vi "dfd_DFXPSimu Casting (vector).vi"(5 "quantize output? (T)":bool=TRUE, 7 "op params":T3={"source"=0, "is floating?"=FALSE, "o-mode"=enum."Wrap", "q-mode"=enum."Truncation", "wl"=1, "high limit"=0, "low limit"=0, "iwl"=0, "sign?"=TRUE} {"source" items=["Coef a/k"=0, "Coef b/v"=7, "Input"=1, "Output"=2, "Multiplicand"=3, "Product"=4, "Sum"=5, "Delay"=6, "Gain"=8]}, 8 "filtering statistics in":T7(array[cluster]) {"statistics information"."min value" format="%.2f"; "statistics information"."max value" format="%.2f"; "Quantizer Source" items=["Coefficients a/k"=0, "Coefficients b/v"=7, "Input"=1, "Output"=2, "Multiplicand"=3, "Product"=4, "Sum"=5, "Delay"=6]}, 11 "Value in":T8 {"High 64" format="%.0x"; "Low 64" format="%.0x"}) -> (0 "filtering statistics out":T7(array[cluster]) {"statistics information"."min value" format="%.2f"; "statistics information"."max value" format="%.2f"; "Quantizer Source" items=["Coefficients a/k"=0, "Coefficients b/v"=7, "Input"=1, "Output"=2, "Multiplicand"=3, "Product"=4, "Sum"=5, "Delay"=6]}, 3 "Value out":T2)   [LabVIEW 2017, in "NI_DigFilter_FXP.lvlib"]
uses:
  <vilib>/addons/Digital Filter Design/NI_DigFilter_FXP.lvlib
  <vilib>/addons/Digital Filter Design/_Objects.llb/dfd_DFXP Data Type 128bits (vector).ctl
  <vilib>/addons/Digital Filter Design/_Objects.llb/dfd_DFXP Data Type (vector).ctl
  <vilib>/addons/Digital Filter Design/_Objects.llb/DFD Quantization Sources.ctl
  <vilib>/addons/Digital Filter Design/_Objects.llb/DFD FXP Statistics Data.ctl
  <vilib>/addons/Digital Filter Design/_Objects.llb/dfd_DFXP Operation Parameter.ctl
  <vilib>/addons/Digital Filter Design/_Objects.llb/dfd_Internal Quantization Srcs.ctl
  <vilib>/addons/Digital Filter Design/_Objects.llb/dfd_DFXP Data Type 128bits (scaler).ctl
  <vilib>/addons/Digital Filter Design/NI_DigFilterLicensed.lvlib
panel:
  in  "Value type":T1 {"Low 64" format="%.0x"; "High 64" format="%.0x"}
  in  "Value out type":T2
  in  "Value out type":T2
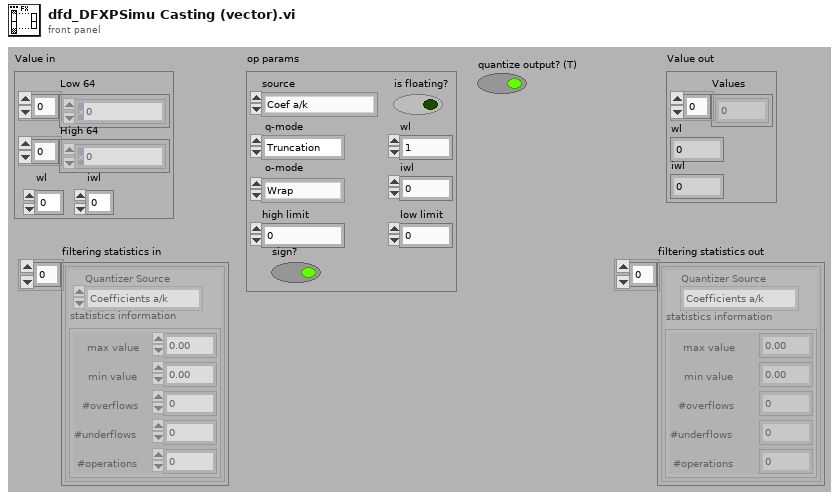
[diagram p1: front panel]
types:
  T1 = typedef "dfd_DFXP Data Type 128bits (scaler).ctl" = cluster{"Low 64":u64, "High 64":i64, "wl":i16, "iwl":i16}
  T2 = typedef "dfd_DFXP Data Type (vector).ctl" = cluster{"Values":i64[], "wl":i16, "iwl":i16}
  T3 = typedef "dfd_DFXP Operation Parameter.ctl" = cluster{"source":T4, "is floating?":bool, "o-mode":enum16{"Saturation", "Wrap"}, "q-mode":enum16{"Nearest", "Truncation"}, "wl":i16, "high limit":i64, "low limit":i64, "iwl":i16, "sign?":bool}
  T4 = typedef "NI_DigFilterLicensed.lvlib/dfd_Internal Quantization Srcs.ctl" = u16
  T5 = typedef "NI_DigFilterLicensed.lvlib/DFD Quantization Sources.ctl" = u16
  T6 = typedef "NI_DigFilterLicensed.lvlib/DFD FXP Statistics Data.ctl" = cluster{"max value":ext, "min value":ext, "#overflows":i32, "#underflows":i32, "#operations":i32}
  T7 = cluster{"Quantizer Source":T5, "statistics information":T6}[]
  T8 = typedef "dfd_DFXP Data Type 128bits (vector).ctl" = cluster{"Low 64":u64[], "High 64":i64[], "wl":i16, "iwl":i16}
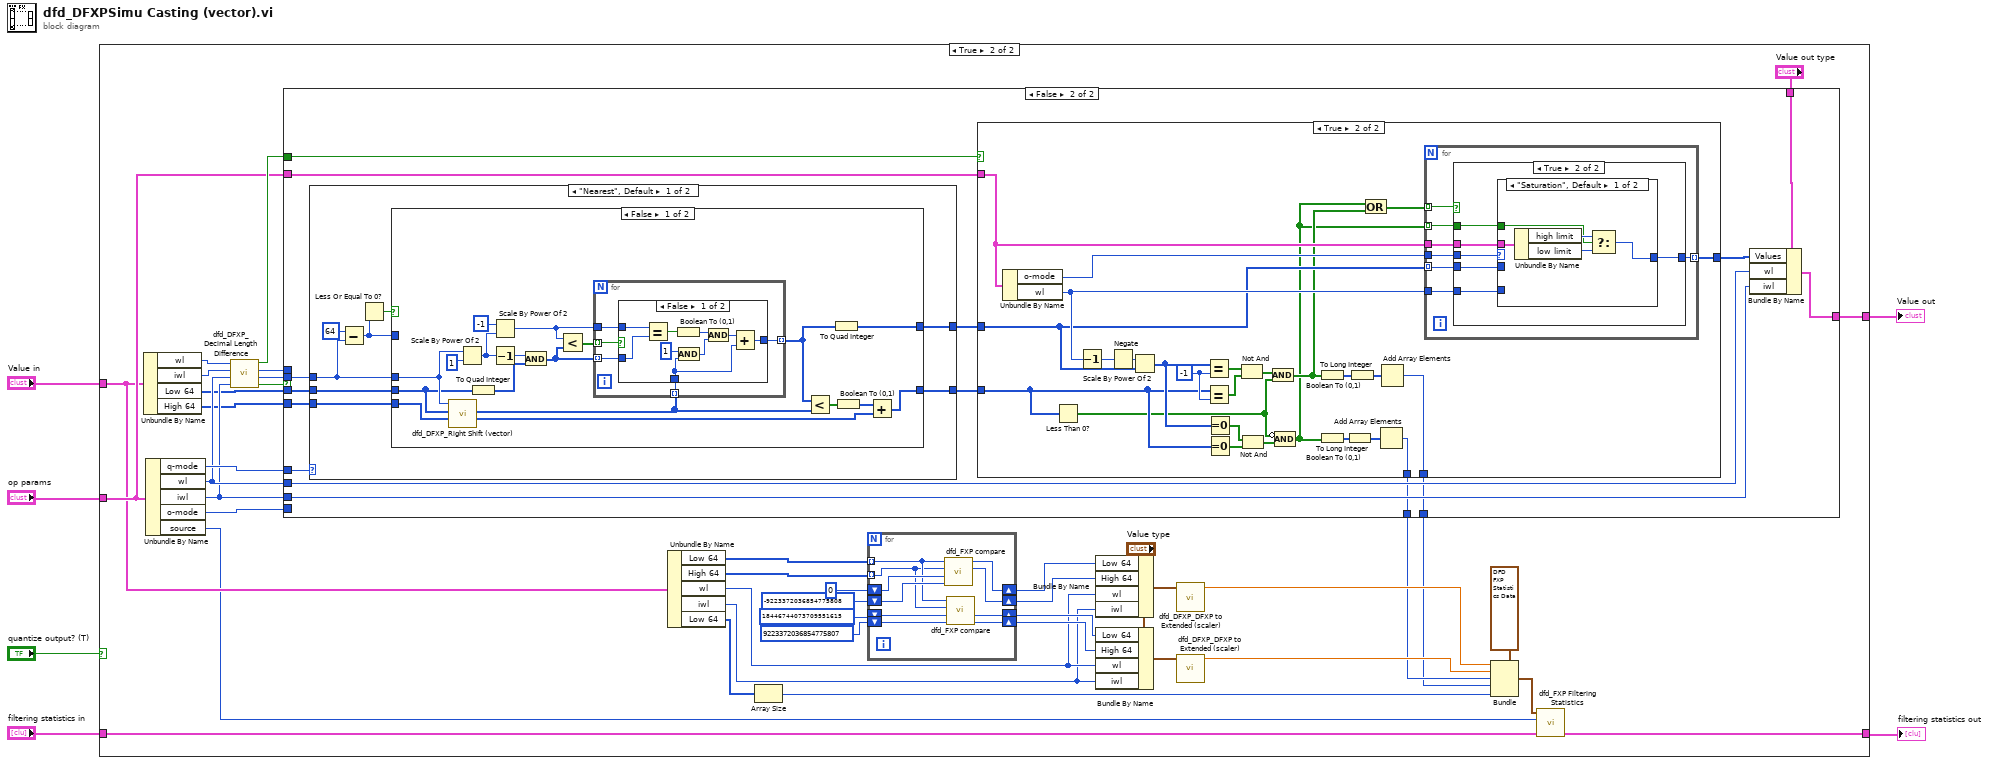
[diagram p0: block diagram]
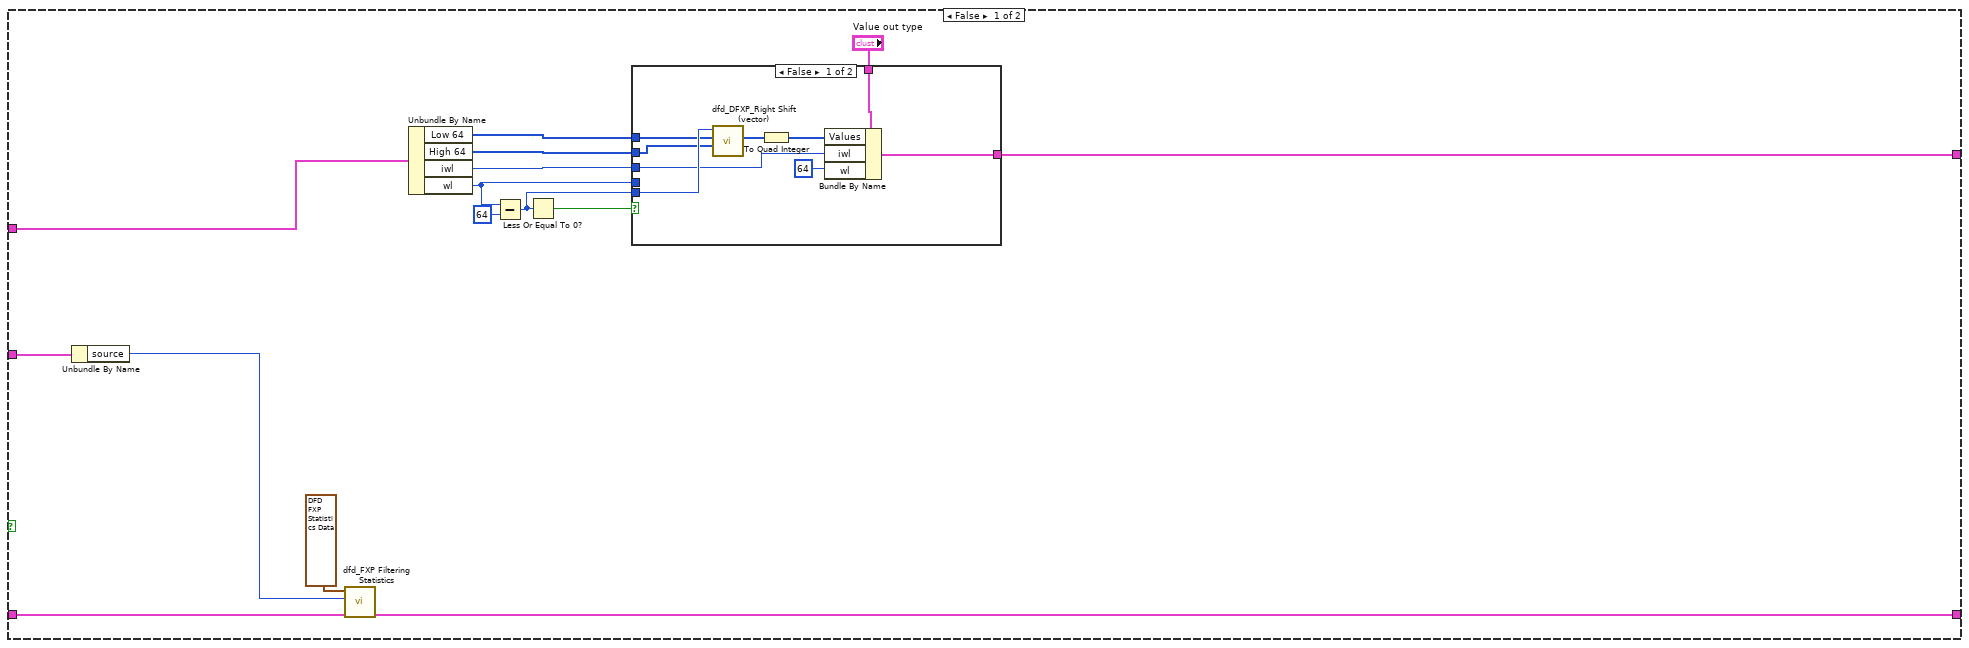
[diagram p2: hidden frame]
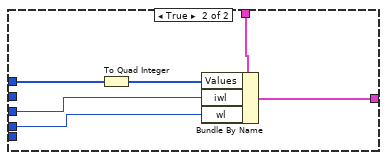
[diagram p3: hidden frame]
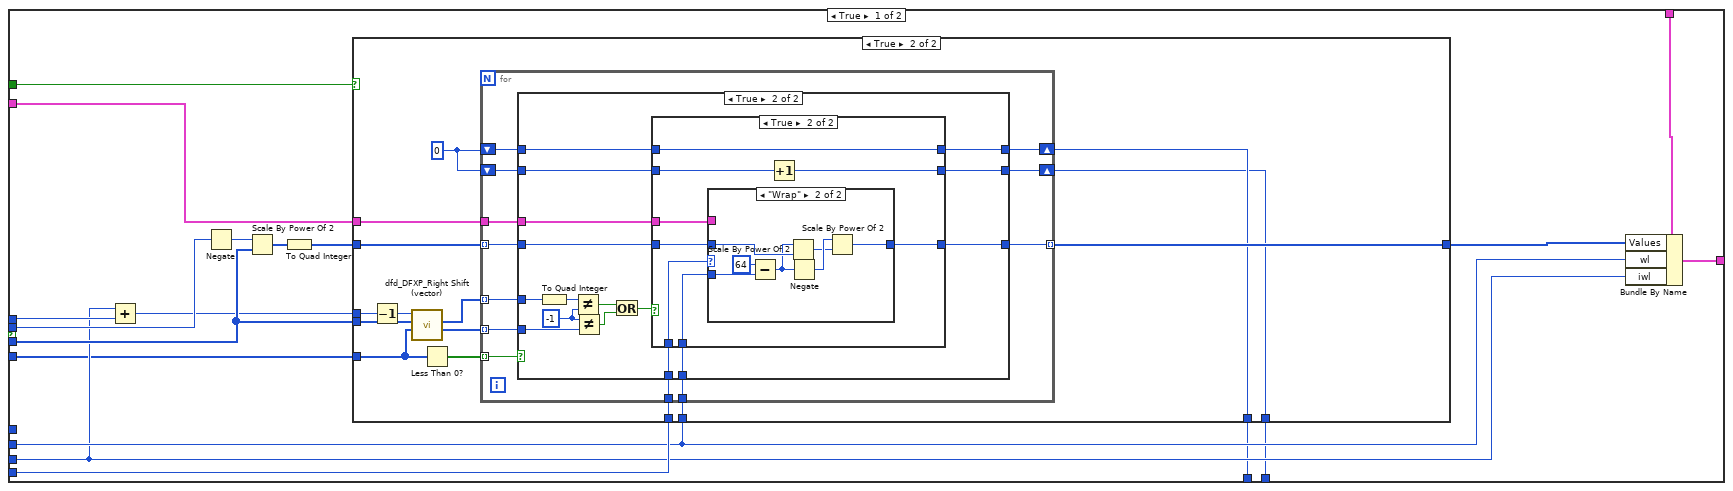
[diagram p4: hidden frame]
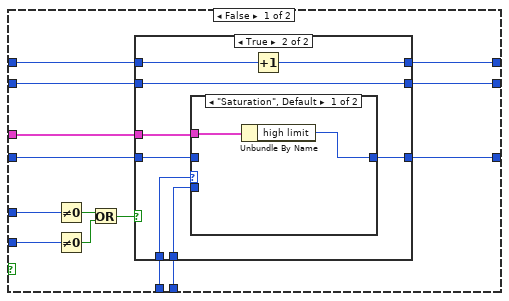
[diagram p6: hidden frame]
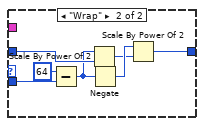
[diagram p8: hidden frame]
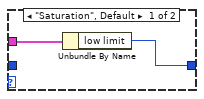
[diagram p10: hidden frame]
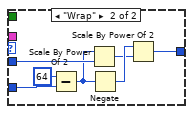
[diagram p13: hidden frame]
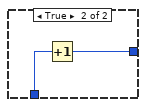
[diagram p14: hidden frame]
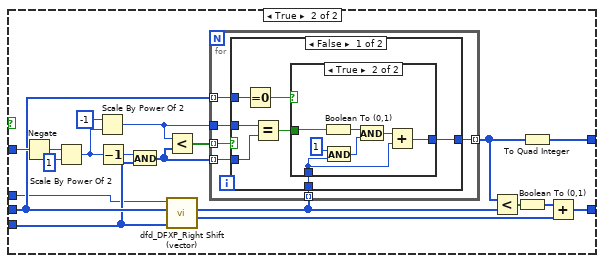
[diagram p15: hidden frame]
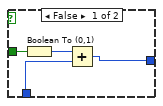
[diagram p16: hidden frame]
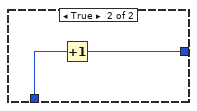
[diagram p17: hidden frame]
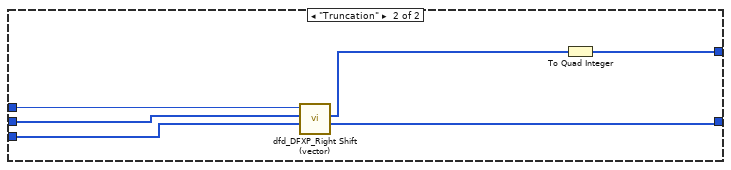
[diagram p18: hidden frame]
diagram:
  n1 = case shown="True" "quantize output? (T)" {
    tunnel: [w12 w67] -> w1
    tunnel: "op params" -> [w21 w70]
    tunnel: "Value in" -> [w13 w63]
    tunnel: "filtering statistics in" -> [w8 w45]
    tunnel: [w7 w37] -> w6
    frame False {
      n2 = Unbundle By Name(w21) -> ("source"=w10:T4)
      n3 = call <vilib>:"dfd_FXP Filtering Statistics.vi"("filtering statistics in"=w8, "source"=w10, "new data"=T6 {"max value"=-inf, "min value"=inf, "#overflows"=0, "#underflows"=0, "#operations"=1}) -> ("filtering statistics out"=w7:T7)  [unwired: 8 in]
      n4 = Unbundle By Name(w13) -> ("Low 64"=w19:u64[], "High 64"=w17:i64[], "iwl"=w18:i16, "wl"=w15:i16)
      n5 = Subtract(x=w15, y=i16 64) -> (x-y=w16:i16)
      n6 = Less Or Equal To 0?(x=w16) -> (x <= 0?=w11:bool)
      n7 = case shown="False" w11 {
        tunnel: w19 -> [w29 w36]
        tunnel: w18 -> [w25 w34]
        tunnel: [w23 w33] -> w12
        tunnel: w17 -> [w28 _]
        tunnel: w16 -> [w30 _]
        tunnel: w15 -> [_ w32]
        tunnel: "Value out type" -> [w22 w31]
        frame False {
          n8 = call <vilib>:"dfd_DFXP_Right Shift (vector).vi"("High 64"=w28, "Low 64"=w29, "Num"=w30) -> ("Low 64"=w26:u64[])  [unwired: 8 out]
          n9 = To Quad Integer(1:w26) -> (0:w27:i64[])
          n10 = Bundle By Name(cluster=w22, "Values"=w27, "iwl"=w25, "wl"=i16 64) -> (w23:T2)
        }
        frame True {
          n11 = To Quad Integer(1:w36) -> (0:w35:i64[])
          n12 = Bundle By Name(cluster=w31, "Values"=w35, "iwl"=w34, "wl"=w32) -> (w33:T2)
        }
      }
    }
    frame True {
      n13 = Unbundle By Name(w63) -> ("wl"=w76:i16, "iwl"=w77:i16, "Low 64"=w66:u64[], "High 64"=w65:i64[])
      n14 = Unbundle By Name(w70) -> ("q-mode"=w78:enum16{"Nearest", "Truncation"}, "wl"=w71:i16, "iwl"=w69:i16, "o-mode"=w72:enum16{"Saturation", "Wrap"}, "source"=w62:T4)
      n15 = call <vilib>:"dfd_DFXP_Decimal Length Difference.vi"("iwl 2"=w69, "wl 2"=w71, "iwl 1"=w77, "wl 1"=w76) -> ("fwl_diff <= 0?"=w75:bool, "fwl_diff"=w73:i16, "fwl"=w64:i16, "iwl_diff >= 0?"=w74:bool)  [unwired: 4 out]
      n16 = case shown="False" w75 {
        tunnel: w78 -> [_ w219]
        tunnel: w66 -> [w97 w218]
        tunnel: w70 -> [w105 w214]
        tunnel: w74 -> [w98 w216]
        tunnel: w73 -> [w96 w215]
        tunnel: w72 -> [w104 _]
        tunnel: w71 -> [w100 w211]
        tunnel: [w99 w209] -> w67
        tunnel: w69 -> [w93 w210]
        tunnel: "Value out type" -> [w102 w213]
        tunnel: w65 -> [w91 w208]
        tunnel: w64 -> [w94 _]
        tunnel: [w90 w206] -> w41
        tunnel: [w89 w205] -> w40
        frame True {
          n17 = Add(x=w93, y=w94) -> (x+y=w92:i16)
          n18 = Negate(x=w96) -> (-x=w106:i16)
          n19 = Scale By Power Of 2(n=w106, x=w97) -> (x*2^n=w103:u64[])
          n20 = To Quad Integer(1:w103) -> (0:w95:i64[])
          n21 = case shown="True" w98 {
            tunnel: w105 -> [_ w115]
            tunnel: w104 -> [_ w114]
            tunnel: w95 -> [w107 w113]
            tunnel: [w107 w111] -> w101
            tunnel: w100 -> [_ w112]
            tunnel: w97 -> [_ w121]
            tunnel: [_ w109] -> w90
            tunnel: [_ w108] -> w89
            tunnel: w92 -> [_ w122]
            tunnel: w91 -> [_ w120]
            frame False {
            }
            frame True {
              w110 = 0 ("high limit")
              n22 = Decrement(x=w122) -> (x-1=w117:i16)
              n23 = call <vilib>:"dfd_DFXP_Right Shift (vector).vi"("High 64"=w120, "Low 64"=w121, "Num"=w117) -> ("High 64"=w118:i64[], "Low 64"=w119:u64[])  [unwired: 7 out]
              n24 = Less Than 0?(x=w120) -> (x < 0?=w116:bool[])
              n25 = for {
                tunnel: w119 -> [w134] mode=indexing
                tunnel: w118 -> [w133] mode=indexing
                tunnel: w116 -> [w132] mode=indexing
                tunnel: w115 -> [w131]
                tunnel: w114 -> [w130]
                tunnel: w113 -> [w129] mode=indexing
                tunnel: w112 -> [w128]
                tunnel: [w127] -> w111 mode=indexing
                shift-right: [w125] -> w109
                shift-left: w110 -> [w126]
                shift-right: [w123] -> w108
                shift-left: w110 -> [w124]
                n26 = case shown="True" w132 {
                  tunnel: w134 -> [w148 w181]
                  tunnel: w133 -> [w147 w180]
                  tunnel: w131 -> [w143 w173]
                  tunnel: w130 -> [w142 w170]
                  tunnel: w129 -> [w141 w172]
                  tunnel: w128 -> [w140 w171]
                  tunnel: [w139 w169] -> w127
                  tunnel: w126 -> [w138 w177]
                  tunnel: [w137 w175] -> w125
                  tunnel: w124 -> [w136 w176]
                  tunnel: [w135 w174] -> w123
                  frame False {
                    n27 = Not Equal To 0?(x=w148) -> (x != 0?=w146:bool)
                    n28 = Not Equal To 0?(x=w147) -> (x != 0?=w145:bool)
                    n29 = Or(x=w146, y=w145) -> (x .or. y?=w144:bool)
                    n30 = case shown="True" w144 {
                      tunnel: [w151 w159] -> w139
                      tunnel: w141 -> [w151 w158]
                      tunnel: w143 -> [_ w157]
                      tunnel: w142 -> [_ w156]
                      tunnel: w140 -> [_ w155]
                      tunnel: w138 -> [w150 w154]
                      tunnel: [w150 w153] -> w137
                      tunnel: w136 -> [w149 w152]
                      tunnel: [w149 w152] -> w135
                      frame False {
                      }
                      frame True {
                        n31 = case shown="\"Saturation\", Default" w156 {
                          tunnel: [w160 w167] -> w159
                          tunnel: w155 -> [_ w168]
                          tunnel: w158 -> [_ w166]
                          tunnel: w157 -> [w161 _]
                          frame "Saturation", Default {
                            n32 = Unbundle By Name(w161) -> ("high limit"=w160:i64)
                          }
                          frame "Wrap" {
                            n33 = Subtract(x=i16 64, y=w168) -> (x-y=w164:i16)
                            n34 = Scale By Power Of 2(n=w164, x=w166) -> (x*2^n=w162:i64)
                            n35 = Negate(x=w164) -> (-x=w163:i16)
                            n36 = Scale By Power Of 2(n=w163, x=w162) -> (x*2^n=w167:i64)
                          }
                        }
                        n37 = Increment(x=w154) -> (x+1=w153:i32)
                      }
                    }
                  }
                  frame True {
                    w183 = i64 -1 ("y")
                    n38 = To Quad Integer(1:w181) -> (0:w179:i64)
                    n39 = Not Equal?(x=w179, y=w183) -> (x != y?=w184:bool)
                    n40 = Not Equal?(x=w183, y=w180) -> (x != y?=w182:bool)
                    n41 = Or(x=w184, y=w182) -> (x .or. y?=w178:bool)
                    n42 = case shown="True" w178 {
                      tunnel: [w187 w195] -> w169
                      tunnel: w172 -> [w187 w194]
                      tunnel: w173 -> [_ w193]
                      tunnel: w170 -> [_ w192]
                      tunnel: w171 -> [_ w191]
                      tunnel: w177 -> [w186 w189]
                      tunnel: [w186 w189] -> w175
                      tunnel: w176 -> [w185 w190]
                      tunnel: [w185 w188] -> w174
                      frame False {
                      }
                      frame True {
                        n43 = case shown="\"Wrap\"" w192 {
                          tunnel: [w196 w203] -> w195
                          tunnel: w191 -> [_ w204]
                          tunnel: w194 -> [_ w202]
                          tunnel: w193 -> [w197 _]
                          frame "Saturation", Default {
                            n44 = Unbundle By Name(w197) -> ("low limit"=w196:i64)
                          }
                          frame "Wrap" {
                            n45 = Subtract(x=i16 64, y=w204) -> (x-y=w200:i16)
                            n46 = Scale By Power Of 2(n=w200, x=w202) -> (x*2^n=w198:i64)
                            n47 = Negate(x=w200) -> (-x=w199:i16)
                            n48 = Scale By Power Of 2(n=w199, x=w198) -> (x*2^n=w203:i64)
                          }
                        }
                        n49 = Increment(x=w190) -> (x+1=w188:i32)
                      }
                    }
                  }
                }
              }
            }
          }
          n50 = Bundle By Name(cluster=w102, "Values"=w101, "wl"=w100, "iwl"=w93) -> (w99:T2)
        }
        frame False {
          n51 = case shown="\"Nearest\", Default" w219 {
            tunnel: w215 -> [w278 w365]
            tunnel: w218 -> [w279 w364]
            tunnel: [w277 w360] -> w217
            tunnel: w208 -> [w276 w363]
            tunnel: [w273 w361] -> w207
            frame "Nearest", Default {
              n52 = Subtract(x=i16 64 ("y"), y=w278) -> (x-y=w274:i16)
              n53 = Less Or Equal To 0?(x=w274) -> (x <= 0?=w275:bool)
              n54 = case shown="False" w275 {
                tunnel: w279 -> [w290 w324]
                tunnel: w278 -> [w291 w322]
                tunnel: [w281 w315] -> w277
                tunnel: w276 -> [w289 w323]
                tunnel: w274 -> [_ w326]
                tunnel: [w283 w316] -> w273
                frame False {
                  n55 = call <vilib>:"dfd_DFXP_Right Shift (vector).vi"("High 64"=w289, "Low 64"=w290, "Num"=w291) -> ("High 64"=w284:i64[], "Low 64"=w287:u64[])  [unwired: 7 out]
                  n56 = Scale By Power Of 2(n=w291, x=i64 1) -> (x*2^n=w295:i64)
                  n57 = To Quad Integer(1:w290) -> (0:w288:i64[])
                  n58 = Scale By Power Of 2(n=-1, x=w295) -> (x*2^n=w296:i64)
                  n59 = Decrement(x=w295) -> (x-1=w293:i64)
                  n60 = And(x=w293, y=w288) -> (x .and. y?=w297:i64[])
                  n61 = Less?(x=w296, y=w297) -> (x < y?=w298:bool[])
                  n62 = for {
                    tunnel: w298 -> [w303] mode=indexing
                    tunnel: w297 -> [w302] mode=indexing
                    tunnel: w296 -> [w301]
                    tunnel: w287 -> [w300] mode=indexing
                    tunnel: [w299] -> w282 mode=indexing
                    n63 = case shown="False" w303 {
                      tunnel: w301 -> [w312 _]
                      tunnel: w302 -> [w311 _]
                      tunnel: w300 -> [w304 w314]
                      tunnel: [w306 w313] -> w299
                      frame False {
                        n64 = Equal?(x=w312, y=w311) -> (x = y?=w309:bool)
                        n65 = Boolean To (0,1)(Boolean=w309) -> (0, 1=w308:i16)
                        n66 = And(x=u64 1, y=w304) -> (x .and. y?=w307:u64)
                        n67 = And(x=w308, y=w307) -> (x .and. y?=w305:u64)
                        n68 = Add(x=w305, y=w304) -> (x+y=w306:u64)
                      }
                      frame True {
                        n69 = Increment(x=w314) -> (x+1=w313:u64)
                      }
                    }
                  }
                  n70 = Less?(x=w282, y=w287) -> (x < y?=w286:bool[])
                  n71 = To Quad Integer(1:w282) -> (0:w281:i64[])
                  n72 = Boolean To (0,1)(Boolean=w286) -> (0, 1=w285:i16[])
                  n73 = Add(x=w285, y=w284) -> (x+y=w283:i64[])
                }
                frame True {
                  n74 = Negate(x=w326) -> (-x=w325:i16)
                  n75 = Scale By Power Of 2(n=w325, x=i64 1) -> (x*2^n=w330:i64)
                  n76 = Scale By Power Of 2(n=-1, x=w330) -> (x*2^n=w329:i64)
                  n77 = Decrement(x=w330) -> (x-1=w332:i64)
                  n78 = And(x=w332, y=w323) -> (x .and. y?=w328:i64[])
                  n79 = Less?(x=w329, y=w328) -> (x < y?=w327:bool[])
                  n80 = call <vilib>:"dfd_DFXP_Right Shift (vector).vi"("High 64"=w323, "Low 64"=w324, "Num"=w322) -> ("High 64"=w317:i64[], "Low 64"=w320:u64[])  [unwired: 7 out]
                  n81 = for {
                    tunnel: w329 -> [w339]
                    tunnel: w328 -> [w338] mode=indexing
                    tunnel: w327 -> [w337] mode=indexing
                    tunnel: w324 -> [w336] mode=indexing
                    tunnel: [w335] -> w321 mode=indexing
                    tunnel: w320 -> [w334] mode=indexing
                    n82 = case shown="False" w337 {
                      tunnel: w339 -> [w346 _]
                      tunnel: w338 -> [w345 _]
                      tunnel: w334 -> [w341 w359]
                      tunnel: [w340 w358] -> w335
                      tunnel: w336 -> [w344 _]
                      frame False {
                        n83 = Equal To 0?(x=w344) -> (x = 0?=w343:bool)
                        n84 = Equal?(x=w346, y=w345) -> (x = y?=w342:bool)
                        n85 = case shown="True" w343 {
                          tunnel: w342 -> [w350 w353]
                          tunnel: w341 -> [w348 w352]
                          tunnel: [w347 w351] -> w340
                          frame False {
                            n86 = Boolean To (0,1)(Boolean=w350) -> (0, 1=w349:i16)
                            n87 = Add(x=w349, y=w348) -> (x+y=w347:u64)
                          }
                          frame True {
                            n88 = Boolean To (0,1)(Boolean=w353) -> (0, 1=w355:i16)
                            n89 = And(x=u64 1, y=w352) -> (x .and. y?=w356:u64)
                            n90 = And(x=w355, y=w356) -> (x .and. y?=w357:u64)
                            n91 = Add(x=w357, y=w352) -> (x+y=w351:u64)
                          }
                        }
                      }
                      frame True {
                        n92 = Increment(x=w359) -> (x+1=w358:u64)
                      }
                    }
                  }
                  n93 = Less?(x=w321, y=w320) -> (x < y?=w319:bool[])
                  n94 = Boolean To (0,1)(Boolean=w319) -> (0, 1=w318:i16[])
                  n95 = To Quad Integer(1:w321) -> (0:w315:i64[])
                  n96 = Add(x=w318, y=w317) -> (x+y=w316:i64[])
                }
              }
            }
            frame "Truncation" {
              n97 = call <vilib>:"dfd_DFXP_Right Shift (vector).vi"("High 64"=w363, "Low 64"=w364, "Num"=w365) -> ("High 64"=w361:i64[], "Low 64"=w362:u64[])  [unwired: 7 out]
              n98 = To Quad Integer(1:w362) -> (0:w360:i64[])
            }
          }
          n99 = case shown="True" w216 {
            tunnel: w217 -> [w220 w234]
            tunnel: w214 -> [_ w244]
            tunnel: [w220 w243] -> w212
            tunnel: [_ w237] -> w206
            tunnel: [_ w238] -> w205
            tunnel: w207 -> [_ w227]
            frame False {
            }
            frame True {
              w231 = i64 -1 ("y")
              n100 = Unbundle By Name(w244) -> ("o-mode"=w245:enum16{"Saturation", "Wrap"}, "wl"=w235:i16)
              n101 = Less Than 0?(x=w227) -> (x < 0?=w223:bool[])
              n102 = Decrement(x=w235) -> (x-1=w221:i16)
              n103 = Negate(x=w221) -> (-x=w236:i16)
              n104 = Scale By Power Of 2(n=w236, x=w234) -> (x*2^n=w228:i64[])
              n105 = Equal?(x=w228, y=w231) -> (x = y?=w230:bool[])
              n106 = Equal?(x=w227, y=w231) -> (x = y?=w229:bool[])
              n107 = Equal To 0?(x=w228) -> (x = 0?=w233:bool[])
              n108 = Equal To 0?(x=w227) -> (x = 0?=w232:bool[])
              n109 = Not And(1:w229, 2:w230) -> (0:w226:bool[])
              n110 = Not And(1:w232, 2:w233) -> (0:w224:bool[])
              n111 = And(x=w226, y=w223) -> (x .and. y?=w225:bool[])
              n112 = Compound Arithmetic op=AND(invert w223, w224) -> (w222:bool[])
              n113 = Boolean To (0,1)(Boolean=w225) -> (0, 1=w242:i16[])
              n114 = Boolean To (0,1)(Boolean=w222) -> (0, 1=w241:i16[])
              n115 = To Long Integer(number=w241) -> (32bit integer=w239:i32[])
              n116 = To Long Integer(number=w242) -> (32bit integer=w240:i32[])
              n117 = Compound Arithmetic op=OR(w222, w225) -> (w246:bool[])
              n118 = Add Array Elements(numeric array=w239) -> (sum=w237:i32)
              n119 = Add Array Elements(numeric array=w240) -> (sum=w238:i32)
              n120 = for {
                tunnel: w246 -> [w253] mode=indexing
                tunnel: w245 -> [w252]
                tunnel: w235 -> [w251]
                tunnel: w234 -> [w250] mode=indexing
                tunnel: w244 -> [w249]
                tunnel: [w248] -> w243 mode=indexing
                tunnel: w222 -> [w247] mode=indexing
                n121 = case shown="True" w253 {
                  tunnel: w252 -> [_ w260]
                  tunnel: [w254 w259] -> w248
                  tunnel: w251 -> [_ w258]
                  tunnel: w250 -> [w254 w257]
                  tunnel: w249 -> [_ w256]
                  tunnel: w247 -> [_ w255]
                  frame False {
                  }
                  frame True {
                    n122 = case shown="\"Saturation\", Default" w260 {
                      tunnel: [w262 w271] -> w259
                      tunnel: w258 -> [_ w272]
                      tunnel: w257 -> [_ w270]
                      tunnel: w256 -> [w265 _]
                      tunnel: w255 -> [w261 _]
                      frame "Saturation", Default {
                        n123 = Unbundle By Name(w265) -> ("high limit"=w264:i64, "low limit"=w263:i64)
                        n124 = Select(t=w264, s=w261, f=w263) -> (s? t:f=w262:i64)
                      }
                      frame "Wrap" {
                        n125 = Subtract(x=i16 64, y=w272) -> (x-y=w268:i16)
                        n126 = Scale By Power Of 2(n=w268, x=w270) -> (x*2^n=w266:i64)
                        n127 = Negate(x=w268) -> (-x=w267:i16)
                        n128 = Scale By Power Of 2(n=w267, x=w266) -> (x*2^n=w271:i64)
                      }
                    }
                  }
                }
              }
            }
          }
          n129 = Bundle By Name(cluster=w213, "Values"=w212, "wl"=w211, "iwl"=w210) -> (w209:T2)
        }
      }
      n130 = Unbundle By Name(w63) -> ("Low 64"=w61:u64[], "High 64"=w60:i64[], "wl"=w50:i16, "iwl"=w49:i16, "Low 64"=w46:u64[])
      n131 = Array Size(array=w46) -> (size(s)=w39:i32)
      n132 = for {
        tunnel: w61 -> [w84] mode=indexing
        tunnel: w60 -> [w83] mode=indexing
        shift-right: [w87] -> w55
        shift-left: u64 0 ("Bigger low64") -> [w88]
        shift-right: [w86] -> w54
        shift-left: i64 -9223372036854775808 ("Bigger high64") -> [w85]
        shift-right: [w80] -> w52
        shift-left: u64 18446744073709551615 ("Bigger high64") -> [w82]
        shift-right: [w79] -> w51
        shift-left: i64 9223372036854775807 ("Bigger high64") -> [w81]
        n133 = call <vilib>:"dfd_FXP compare.vi"("High 64_2"=w85, "Low 64_2"=w88, "High 64_1"=w83, "Low 64_1"=w84) -> ("Bigger high64"=w86:i64, "Bigger low64"=w87:u64)  [unwired: 6 out]
        n134 = call <vilib>:"dfd_FXP compare.vi"("High 64_2"=w81, "Low 64_2"=w82, "High 64_1"=w83, "Low 64_1"=w84) -> ("Smaller high64"=w79:i64, "Smaller low64"=w80:u64)  [unwired: 6 out]
      }
      n135 = Bundle By Name(cluster="Value type", "Low 64"=w55, "High 64"=w54, "wl"=w50, "iwl"=w49) -> (w48:T1)
      n136 = Bundle By Name(cluster="Value type", "Low 64"=w52, "High 64"=w51, "wl"=w50, "iwl"=w49) -> (w47:T1)
      n137 = call <vilib>:"dfd_DFXP_DFXP to Extended (scaler).vi"("Value in"=w48) -> ("Ext value"=w43:ext)  [unwired: 10 out]
      n138 = call <vilib>:"dfd_DFXP_DFXP to Extended (scaler).vi"("Value in"=w47) -> ("Ext value"=w42:ext)  [unwired: 10 out]
      n139 = Bundle(cluster=T6 {"max value"=-inf, "min value"=inf, "#overflows"=0, "#underflows"=0, "#operations"=1} ("new data"), "max value"=w43, "min value"=w42, "#overflows"=w41, "#underflows"=w40, "#operations"=w39) -> (w38:T6)
      n140 = call <vilib>:"dfd_FXP Filtering Statistics.vi"("filtering statistics in"=w45, "source"=w62, "new data"=w38) -> ("filtering statistics out"=w37:T7)  [unwired: 8 in]
    }
  }
  "Value out" <- w1
  "filtering statistics out" <- w6
